vi "keccak.calc.Bx.vi"(10 "index":i32, 11 "state[24]":u64[](array[numeric])=[0, 0, 0, 0, 0, 0, 0, 0, 0, 0, 0, 0, 0, 0, 0, 0, 0, 0, 0, 0, 0, 0, 0, 0]) -> (3 "Numeric":u64)   [LabVIEW 2021]
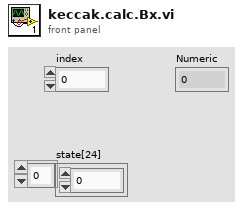
[diagram p1: front panel]
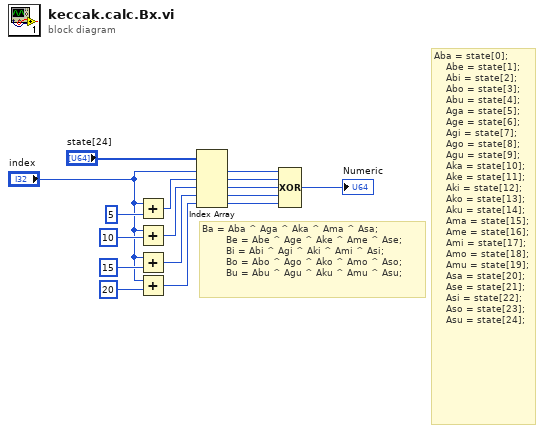
[diagram p0: block diagram]
diagram:
  # "Aba = state[0];\n    Abe = state[1];\n    Abi = state[2];\n    Abo = state[3];\n    Abu = state[4];\n    Aga = state[5];\n    Age = state[6];\n    Agi = state[7];\n    Ago = state[8];\n    Agu = state[9];\n    Aka = state[10];\n    Ake = state[11];\n    Aki = state[12];\n    Ako = state[13];\n    Aku = state[14];\n    Ama = state[15];\n    Ame = state[16];\n    Ami = state[17];\n    Amo = state[18];\n    Amu = state[19];\n    Asa = state[20];\n    Ase = state[21];\n    Asi = state[22];\n    Aso = state[23];\n    Asu = state[24];"
  # "Ba = Aba ^ Aga ^ Aka ^ Ama ^ Asa;\n        Be = Abe ^ Age ^ Ake ^ Ame ^ Ase;\n        Bi = Abi ^ Agi ^ Aki ^ Ami ^ Asi;\n        Bo = Abo ^ Ago ^ Ako ^ Amo ^ Aso;\n        Bu = Abu ^ Agu ^ Aku ^ Amu ^ Asu;"
  n1 = Add(x="index", y=5) -> (x+y=w7:i32)
  n2 = Add(x="index", y=10) -> (x+y=w8:i32)
  n3 = Add(x="index", y=15) -> (x+y=w9:i32)
  n4 = Add(x="index", y=20) -> (x+y=w10:i32)
  n5 = Index Array(array="state[24]", index #1="index", index #2=w7, index #3=w8, index #4=w9, index #5=w10) -> (element #1=w11:u64, element #2=w15:u64, element #3=w14:u64, element #4=w13:u64, element #5=w12:u64)
  n6 = Compound Arithmetic op=XOR(w11, w15, w14, w13, w12) -> (→"Numeric":u64)
